vi "ReadGetFoodQuantity.vi"(8 "error in (no error)":errorcluster, 11 "Duck in":refnum<class "Mouse.lvclass">) -> (0 "error out":errorcluster, 2 "GetFoodQuantity":i32, 3 "Duck out":refnum<class "Mouse.lvclass">)   [LabVIEW 2013, in "Mouse.lvclass"]
uses:
  Mouse.lvclass
  Mouse.lvclass/Mouse.ctl
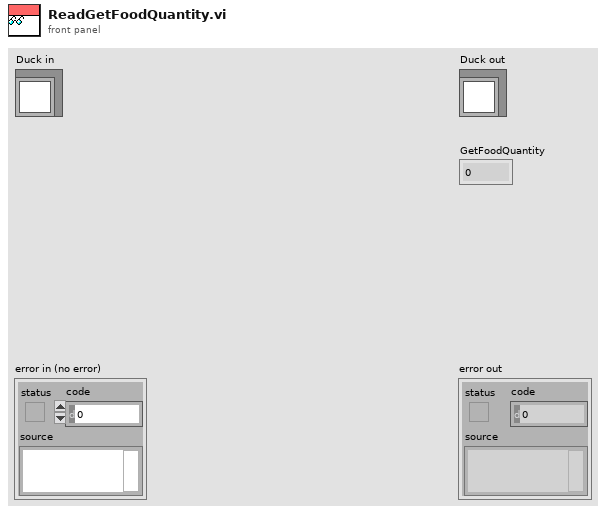
[diagram p1: front panel]
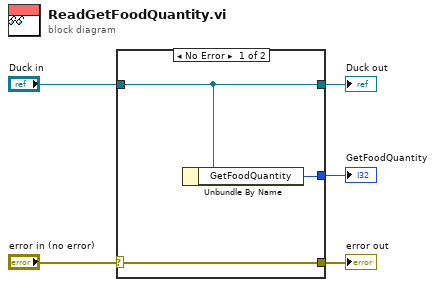
[diagram p0: block diagram]
diagram:
  n1 = case shown="No Error" "error in (no error)" {
    selector: "error in (no error)" -> [w8 w9]
    tunnel: [w8 w9] -> w4
    tunnel: [w6 w10] -> w2
    tunnel: "Duck in" -> [w6 w10]
    tunnel: [w7 _] -> w1
    frame No Error {
      n2 = Unbundle By Name(w6) -> ("GetFoodQuantity"=w7:i32)
    }
    frame Error {
    }
  }
  "error out" <- w4
  "Duck out" <- w2
  "GetFoodQuantity" <- w1
